vi "SG Tests.vi"(8 "error in (no error)":errorcluster) -> (0 "error out":errorcluster)   [LabVIEW 2016]
uses:
  <vilib>/addons/_JKI Toolkits/Caraya/classes/Assert/Assert Almost Equal_Float.vi
  Source/SG/SG.lvlib
  <vilib>/addons/_JKI Toolkits/Caraya/classes/Assert/Assert.lvclass
  <vilib>/addons/_JKI Toolkits/Caraya/classes/Test/Test.lvclass
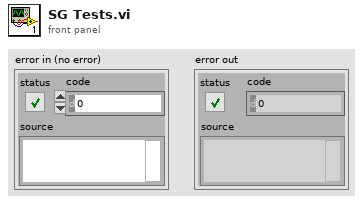
[diagram p1: front panel]
types:
  T1 = typedef "SG.lvlib/Waveform.ctl" = cluster{"Waveform Name":string, "Waveform":cluster{"x0":dbl, "dx":dbl, "y":csg[]}, "Signal Bandwidth (Hz)":dbl, "PAPR (dB)":dbl, "Burst Length (s)":dbl, "Sample Rate":dbl, "Burst Start Locations":i32[], "Burst Stop Locations":i32[], "Idle Duration Present?":bool, "Runtime Scaling":dbl}
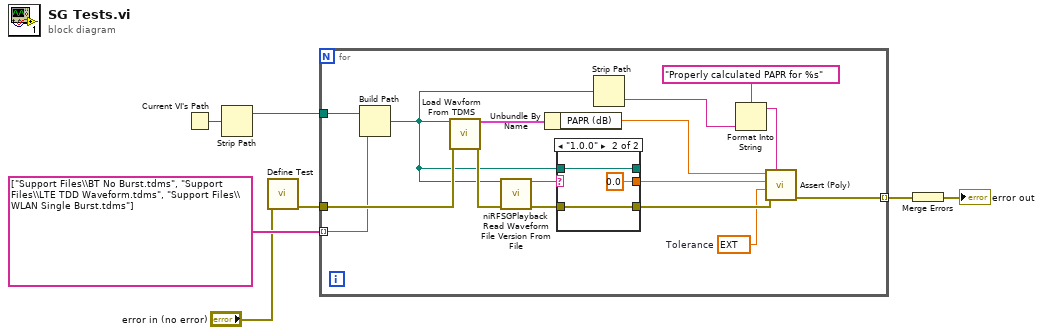
[diagram p0: block diagram]
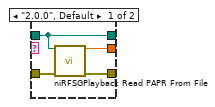
[diagram p2: hidden frame]
diagram:
  n1 = Current VI's Path() -> (path=w7:path)
  n2 = Strip Path(path=w7) -> (stripped path=w6:path)  [unwired: 1 out]
  n3 = call <vilib>:"Define Test.vi"("error in (no error)"="error in (no error)") -> ("error out"=w4:errorcluster)  [unwired: 10 in]
  n4 = for {
    tunnel: w6 -> [w21]
    tunnel: string[] ["Support Files\\BT No Burst.tdms", "Support Files\\LTE TDD Waveform.tdms", "Support Files\\WLAN Single Burst.tdms"] -> [w10] mode=indexing
    tunnel: w4 -> [w23]
    tunnel: [w9] -> w3 mode=indexing
    w11 = ext 0.00099999999999999999996  # Tolerance
    n5 = Build Path(base path=w21, name or relative path=w10) -> (appended path=w8:path)
    n6 = call "Load Wavform From TDMS.vi"("TDMS File Path"=w8, "error in (no error)"=w23) -> ("Waveform"=w17:T1, "error out"=w22:errorcluster)  [unwired: 12 in]
    n7 = call <instrlib>:"niRFSGPlayback Read Waveform File Version From File.vi"("file path"=w8, "error in"=w22) -> ("waveform file version"=w20:string, "error out"=w19:errorcluster)  [unwired: 12 in]
    n8 = Unbundle By Name(w17) -> ("PAPR (dB)"=w16:dbl)
    n9 = case shown="\"1.0.0\"" w20 {
      tunnel: w19 -> [w25 w28]
      tunnel: [w24 w30] -> _
      tunnel: [w27 0.0 ("PAPR")] -> w15
      tunnel: [w26 w28] -> w18
      tunnel: w8 -> [w24 w30]
      frame "2.0.0", Default {
        n10 = call <instrlib>:"niRFSGPlayback Read PAPR From File.vi"("file path"=w24, "error in"=w25) -> ("PAPR"=w27:dbl, "error out"=w26:errorcluster)  [unwired: 12 in]
      }
      frame "1.0.0" {
      }
    }
    n11 = Strip Path(path=w8) -> (name=w13:string)  [unwired: 1 out]
    n12 = Format Into String(format string="Properly calculated PAPR for %s", w13) -> (resulting string=w12:string)  [unwired: 2 in, 1 out]
    n13 = call-poly <vilib>:"Assert (Poly).vi"("Label"=w12, "error in (no error)"=w18, "Tolerance"=w11, "Y"=w15, "X"=w16) -> ("error out"=w9:errorcluster)  [unwired: 6 in]
  }
  n14 = Merge Errors(w3) -> (→"error out":errorcluster)
